vi "Get Valid Decay Fit Parameters List.vi"(1 "Parameter ID Array Size":i32) -> (0 "Current Version":T1[](array[typedef]))   [LabVIEW 2021, in "Fits.lvlib"]
uses:
  Fits.lvlib
  Decay Fit Parameters & Derived Quantities List v2.ctl
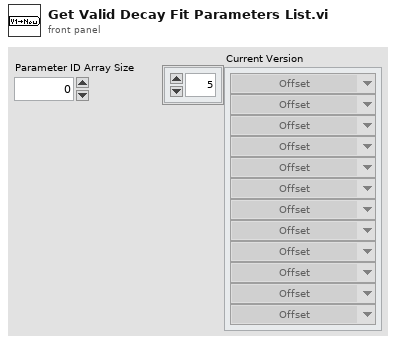
[diagram p1: front panel]
types:
  T1 = typedef "Fits.lvlib/Decay Fit Parameters & Derived Quantities List v2.ctl" = enum16{"Offset", "Baseline", "A_1", "tau_1", "A_2", "tau_2", "<tau>_a", "f1_a", "f2_a", "<tau>_i", "f1_i", "f2_i", "-", "R^2", "Chi^2"}
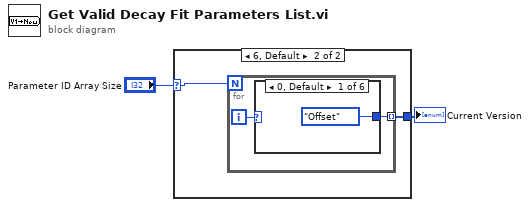
[diagram p0: block diagram]
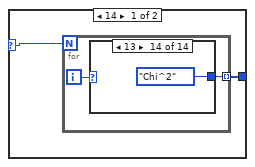
[diagram p2: hidden frame]
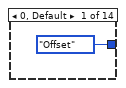
[diagram p3: hidden frame]
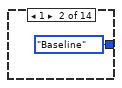
[diagram p4: hidden frame]
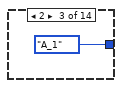
[diagram p5: hidden frame]
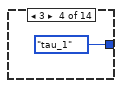
[diagram p6: hidden frame]
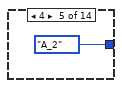
[diagram p7: hidden frame]
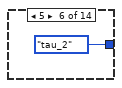
[diagram p8: hidden frame]
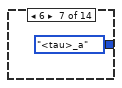
[diagram p9: hidden frame]
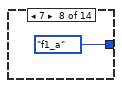
[diagram p10: hidden frame]
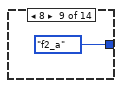
[diagram p11: hidden frame]
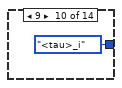
[diagram p12: hidden frame]
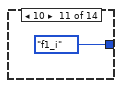
[diagram p13: hidden frame]
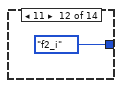
[diagram p14: hidden frame]
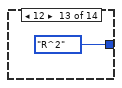
[diagram p15: hidden frame]
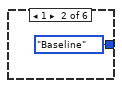
[diagram p16: hidden frame]
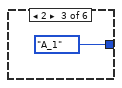
[diagram p17: hidden frame]
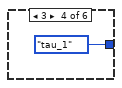
[diagram p18: hidden frame]
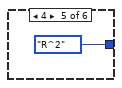
[diagram p19: hidden frame]
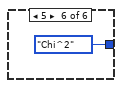
[diagram p20: hidden frame]
diagram:
  n1 = case shown="6, Default" "Parameter ID Array Size" {
    selector: "Parameter ID Array Size" -> [w3 w21]
    tunnel: [w4 w22] -> w2
    frame 14 {
      n2 = for {
        N: w3 -> [_]
        tunnel: [w6] -> w4 mode=indexing
        i -> [w5]
        n3 = case shown="13" w5 {
          tunnel: [Decay_Fit_Parameters_&_Derived_Quantities_List_v2."Offset" ("Current Version") Decay_Fit_Parameters_&_Derived_Quantities_List_v2."Baseline" ("Current Version") Decay_Fit_Parameters_&_Derived_Quantities_List_v2."A_1" ("Current Version") Decay_Fit_Parameters_&_Derived_Quantities_List_v2."tau_1" ("Current Version") Decay_Fit_Parameters_&_Derived_Quantities_List_v2."A_2" ("Current Version") Decay_Fit_Parameters_&_Derived_Quantities_List_v2."tau_2" ("Current Version") Decay_Fit_Parameters_&_Derived_Quantities_List_v2."<tau>_a" ("Current Version") Decay_Fit_Parameters_&_Derived_Quantities_List_v2."f1_a" ("Current Version") Decay_Fit_Parameters_&_Derived_Quantities_List_v2."f2_a" ("Current Version") Decay_Fit_Parameters_&_Derived_Quantities_List_v2."<tau>_i" ("Current Version") Decay_Fit_Parameters_&_Derived_Quantities_List_v2."f1_i" ("Current Version") Decay_Fit_Parameters_&_Derived_Quantities_List_v2."f2_i" ("Current Version") Decay_Fit_Parameters_&_Derived_Quantities_List_v2."R^2" ("Current Version") Decay_Fit_Parameters_&_Derived_Quantities_List_v2."Chi^2" ("Current Version")] -> w6
          frame 0, Default {
          }
          frame 1 {
          }
          frame 2 {
          }
          frame 3 {
          }
          frame 4 {
          }
          frame 5 {
          }
          frame 6 {
          }
          frame 7 {
          }
          frame 8 {
          }
          frame 9 {
          }
          frame 10 {
          }
          frame 11 {
          }
          frame 12 {
          }
          frame 13 {
          }
        }
      }
    }
    frame 6, Default {
      n4 = for {
        N: w21 -> [_]
        tunnel: [w24] -> w22 mode=indexing
        i -> [w23]
        n5 = case shown="0, Default" w23 {
          tunnel: [Decay_Fit_Parameters_&_Derived_Quantities_List_v2."Offset" ("Current Version") Decay_Fit_Parameters_&_Derived_Quantities_List_v2."Baseline" ("Current Version") Decay_Fit_Parameters_&_Derived_Quantities_List_v2."A_1" ("Current Version") Decay_Fit_Parameters_&_Derived_Quantities_List_v2."tau_1" ("Current Version") Decay_Fit_Parameters_&_Derived_Quantities_List_v2."R^2" ("Current Version") Decay_Fit_Parameters_&_Derived_Quantities_List_v2."Chi^2" ("Current Version")] -> w24
          frame 0, Default {
          }
          frame 1 {
          }
          frame 2 {
          }
          frame 3 {
          }
          frame 4 {
          }
          frame 5 {
          }
        }
      }
    }
  }
  "Current Version" <- w2
